vi "Swerve Drive.vi"(5 "Rot. Point X":dbl, 6 "Auto Controls":bool=TRUE, 7 "Rot. Point Y":dbl) -> ()   [LabVIEW 2017]
uses:
  Robot Global Data.vi
panel:
  in  "fr offset":dbl(knob) scale=-180.0..180.0
  in  "fl offset":dbl(knob) scale=-180.0..180.0
  in  "br offset":dbl(knob) scale=-180.0..180.0
  in  "bl offset":dbl(knob) scale=-180.0..180.0
  in  "Robot Length":dbl=24.25
  in  "Robot Width":dbl=21.0
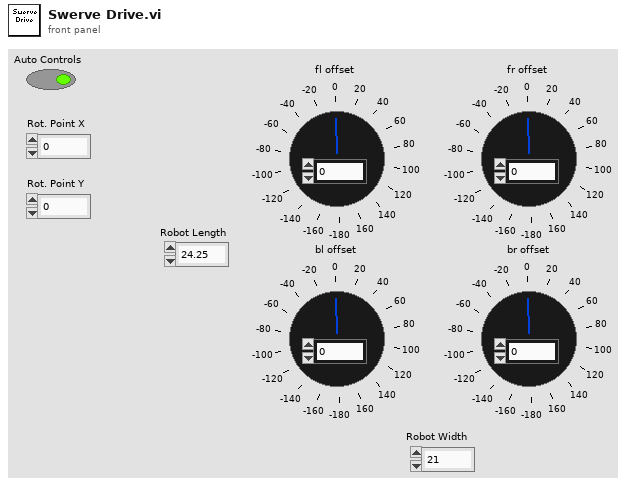
[diagram p1: front panel]
types:
  T1 = enum16{"Back Left", "Back Right", "Front Left", "Front Right"}
  T2 = typedef "WPI_MotorControlDeviceRef.ctl" = cluster{"DeviceStatus":errorcluster, "Type":T3, "PWM":cluster{"PWM Channel":T4, "DeadBand":T5}, "CAN":cluster{"Device Number":u8, "SetOutput VI Ref":variant, "GetOutput VI Ref":variant, "Enable VI Ref":variant, "Disable VI Ref":variant, "Data":variant}, "Invert":bool, "DIO PWM":cluster{"PWM \"Enable\" Channel":T4, "DIOChannel":T6, "PWM Rate":dbl}}
  T3 = typedef "WPI_MotorControlType.ctl" = enum16{"PWM", "CAN", "DIO PWM"}
  T4 = typedef "FPGA_DIOPWMChannel.ctl" = enum8{"PWM 0", "PWM 1", "PWM 2", "PWM 3", "PWM 4", "PWM 5", "PWM 6", "PWM 7", "PWM 8", "PWM 9", "PWM MXP 0", "PWM MXP 1", "PWM MXP 2", "PWM MXP 3", "PWM MXP 4", "PWM MXP 5", "PWM MXP 6", "PWM MXP 7", "PWM MXP 8", "PWM MXP 9", "Invalid"}
  T5 = typedef "WPI_PWMDeadband.ctl" = cluster{"Name":string, "maxPositivePwm":i32, "minPositivePwm":i32, "centerPwm":i32, "maxNegativePwm":i32, "minNegativePwm":i32, "angularRange":u16}
  T6 = typedef "FPGA_DIOChannel.ctl" = enum8{"DIO 0", "DIO 1", "DIO 2", "DIO 3", "DIO 4", "DIO 5", "DIO 6", "DIO 7", "DIO 8", "DIO 9", "DIO MXP 0", "DIO MXP 1", "DIO MXP 2", "DIO MXP 3", "DIO MXP 4", "DIO MXP 5", "DIO MXP 6", "DIO MXP 7", "DIO MXP 8", "DIO MXP 9", "DIO MXP 10", "DIO MXP 11", "DIO MXP 12", "DIO MXP 13", "DIO MXP 14", "DIO MXP 15", "SPI Port CS1", "SPI Port CS2", "SPI Port CS3", "SPI Port MISO", "SPI Port MOSI", "Invalid"}
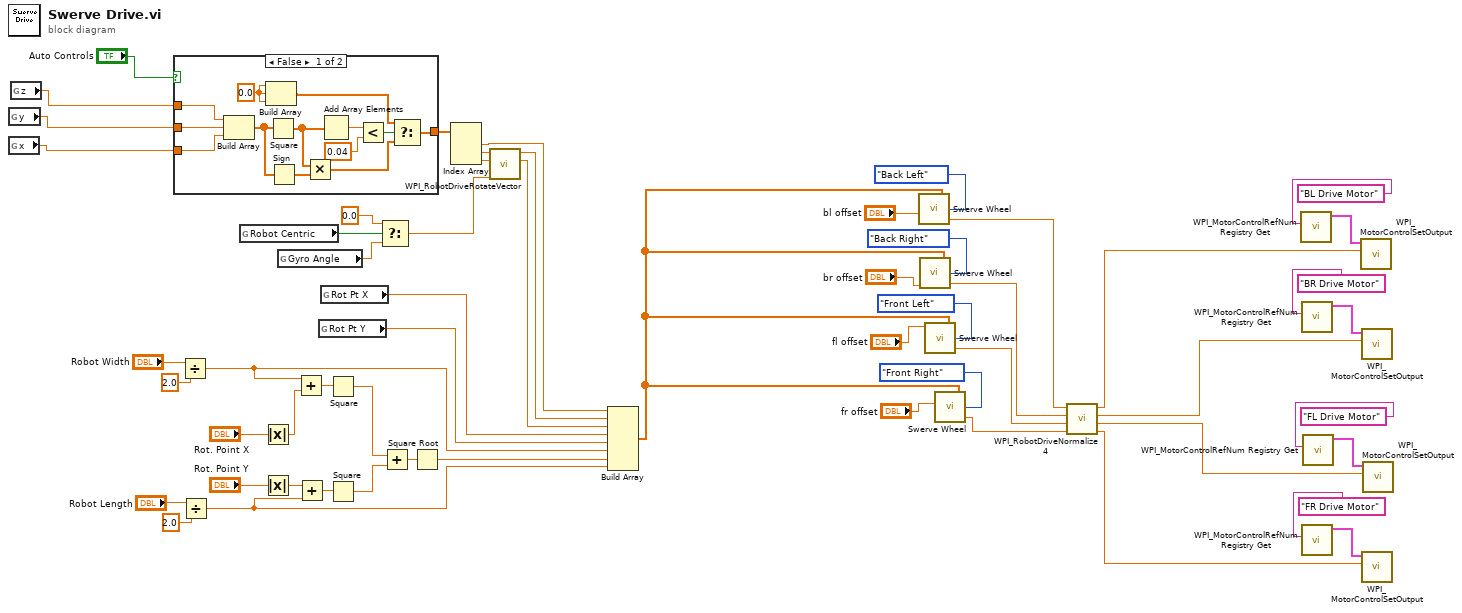
[diagram p0: block diagram]
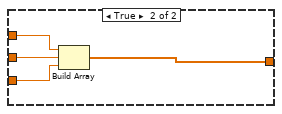
[diagram p2: hidden frame]
diagram:
  n1 = global read "Robot Global Data.vi" "y"() -> (w50:dbl)
  n2 = global read "Robot Global Data.vi" "x"() -> (w53:dbl)
  n3 = global read "Robot Global Data.vi" "z"() -> (w9:dbl)
  n4 = case shown="False" "Auto Controls" {
    tunnel: w50 -> [w58 w73]
    tunnel: w53 -> [w62 w74]
    tunnel: w9 -> [w59 w71]
    tunnel: [w60 w72] -> w52
    frame False {
      w66 = 0.0 ("element")
      n5 = Build Array(w59, w58, w62) -> (w65:dbl[])
      n6 = Build Array(w66, w66, w66) -> (w67:dbl[])
      n7 = Square(x=w65) -> (x^2=w63:dbl[])
      n8 = Sign(1:w65) -> (0:w64:dbl[])
      n9 = Multiply(x=w63, y=w64) -> (x*y=w61:dbl[])
      n10 = Add Array Elements(numeric array=w63) -> (sum=w70:dbl)
      n11 = Less?(x=w70, y=0.04 ("x")) -> (x < y?=w68:bool)
      n12 = Select(t=w67, s=w68, f=w61) -> (s? t:f=w60:dbl[])
    }
    frame True {
      n13 = Build Array(w71, w73, w74) -> (w72:dbl[])
    }
  }
  n14 = Divide(x="Robot Width", y=2.0) -> (x/y=w29:dbl)
  n15 = Divide(x="Robot Length", y=2.0) -> (x/y=w31:dbl)
  n16 = global read "Robot Global Data.vi" "Robot Centric"() -> (w49:bool)
  n17 = Absolute Value(x="Rot. Point X") -> (abs(x)=w43:dbl)
  n18 = Absolute Value(x="Rot. Point Y") -> (abs(x)=w41:dbl)
  n19 = global read "Robot Global Data.vi" "Gyro Angle"() -> (w47:dbl)
  n20 = Add(x=w29, y=w43) -> (x+y=w42:dbl)
  n21 = Add(x=w41, y=w31) -> (x+y=w40:dbl)
  n22 = global read "Robot Global Data.vi" "Rot Pt Y"() -> (w28:dbl)
  n23 = global read "Robot Global Data.vi" "Rot Pt X"() -> (w27:dbl)
  n24 = Square(x=w42) -> (x^2=w38:dbl)
  n25 = Square(x=w40) -> (x^2=w39:dbl)
  n26 = Select(t=0.0, s=w49, f=w47) -> (s? t:f=w44:dbl)
  n27 = Add(x=w38, y=w39) -> (x+y=w37:dbl)
  n28 = Square Root(x=w37) -> (sqrt(x)=w30:dbl)
  n29 = Index Array(array=w52) -> (element #1=w24:dbl, element #2=w46:dbl, element #3=w45:dbl)  [unwired: 3 in]
  n30 = call "WPI_RobotDriveRotateVector.vi"("Angle"=w44, "X"=w45, "Y"=w46) -> ("X'"=w26:dbl, "Y'"=w25:dbl)  [unwired: 7 in]
  n31 = Build Array(w24, w25, w26, w27, w28, w29, w30, w31) -> (w13:dbl[])
  n32 = call "Swerve Wheel.vi"("Wheel"=T1."Back Left", "Inputs"=w13, "bl offset"="bl offset") -> ("Speed"=w21:dbl)  [unwired: 3 in]
  n33 = call "Swerve Wheel.vi"("Wheel"=T1."Back Right", "Inputs"=w13, "br offset"="br offset") -> ("Speed"=w16:dbl)  [unwired: 3 in]
  n34 = call "Swerve Wheel.vi"("Wheel"=T1."Front Left", "Inputs"=w13, "fl offset"="fl offset") -> ("Speed"=w15:dbl)  [unwired: 3 in]
  n35 = call "Swerve Wheel.vi"("Wheel"=T1."Front Right", "Inputs"=w13, "fr offset"="fr offset") -> ("Speed"=w14:dbl)  [unwired: 3 in]
  n36 = call "WPI_RobotDriveNormalize 4.vi"("D"=w14, "C"=w15, "B"=w16, "A"=w21) -> ("D'"=w54:dbl, "C'"=w55:dbl, "B'"=w56:dbl, "A'"=w57:dbl)
  n37 = call <vilib>:"WPI_MotorControlRefNum Registry Get.vi"("refnum name"="BL Drive Motor") -> ("MotorControlDevRef"=w8:T2)  [unwired: 9 in, 1 out]
  n38 = call <vilib>:"WPI_MotorControlRefNum Registry Get.vi"("refnum name"="BR Drive Motor") -> ("MotorControlDevRef"=w7:T2)  [unwired: 9 in, 1 out]
  n39 = call <vilib>:"WPI_MotorControlRefNum Registry Get.vi"("refnum name"="FR Drive Motor") -> ("MotorControlDevRef"=w5:T2)  [unwired: 9 in, 1 out]
  n40 = call <vilib>:"WPI_MotorControlRefNum Registry Get.vi"("refnum name"="FL Drive Motor") -> ("MotorControlDevRef"=w6:T2)  [unwired: 9 in, 1 out]
  n41 = call <vilib>:"WPI_MotorControlSetOutput.vi"("Output"=w57, "MotorControlDevRef"=w8) -> ()  [unwired: 7 in, 3 out]
  n42 = call <vilib>:"WPI_MotorControlSetOutput.vi"("Output"=w56, "MotorControlDevRef"=w7) -> ()  [unwired: 7 in, 3 out]
  n43 = call <vilib>:"WPI_MotorControlSetOutput.vi"("Output"=w54, "MotorControlDevRef"=w5) -> ()  [unwired: 7 in, 3 out]
  n44 = call <vilib>:"WPI_MotorControlSetOutput.vi"("Output"=w55, "MotorControlDevRef"=w6) -> ()  [unwired: 7 in, 3 out]
